vi "OPC UA Client-Write - Multiple Tags.vi"() -> ()   [LabVIEW 2017]
uses:
  <vilib>/OPCUA/controls/NodeId.ctl
  <vilib>/OPCUA/controls/Write Status.ctl
  <vilib>/OPCUA/client/Multiple Write Double Array.vi
  <vilib>/OPCUA/NI OPC UA Client.lvlib
panel:
  out "Temperature Data":dbl[](array[numeric])
  in  "Node Id":string="Process Data.Temperature"
  in  "Stop Button":bool
  in  "Server Endpoint URL":string="opc.tcp://XPS15HPH:49580"
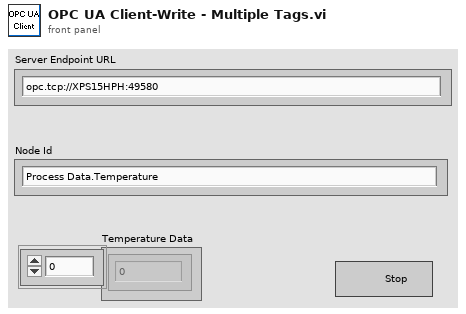
[diagram p1: front panel]
types:
  T1 = cluster{"message mode":enum16{"None", "Sign", "Sign and Encrypt"}, "security":enum16{"Basic256", "Basic128Rsa15"}}
  T2 = typedef "OPC UA Client Refnum.ctl" = refnum<k21>
  T3 = typedef "NodeId.ctl" = string
  T4 = typedef "Write Status.ctl" = u32
  T5 = cluster{"node ID":T3, "value":dbl[], "timestamp (current time)":timestamp, "node status":T4}
  T6 = cluster{"node ID":T3, "value":dbl[], "timestamp (current time)":timestamp, "node status":T4}[]
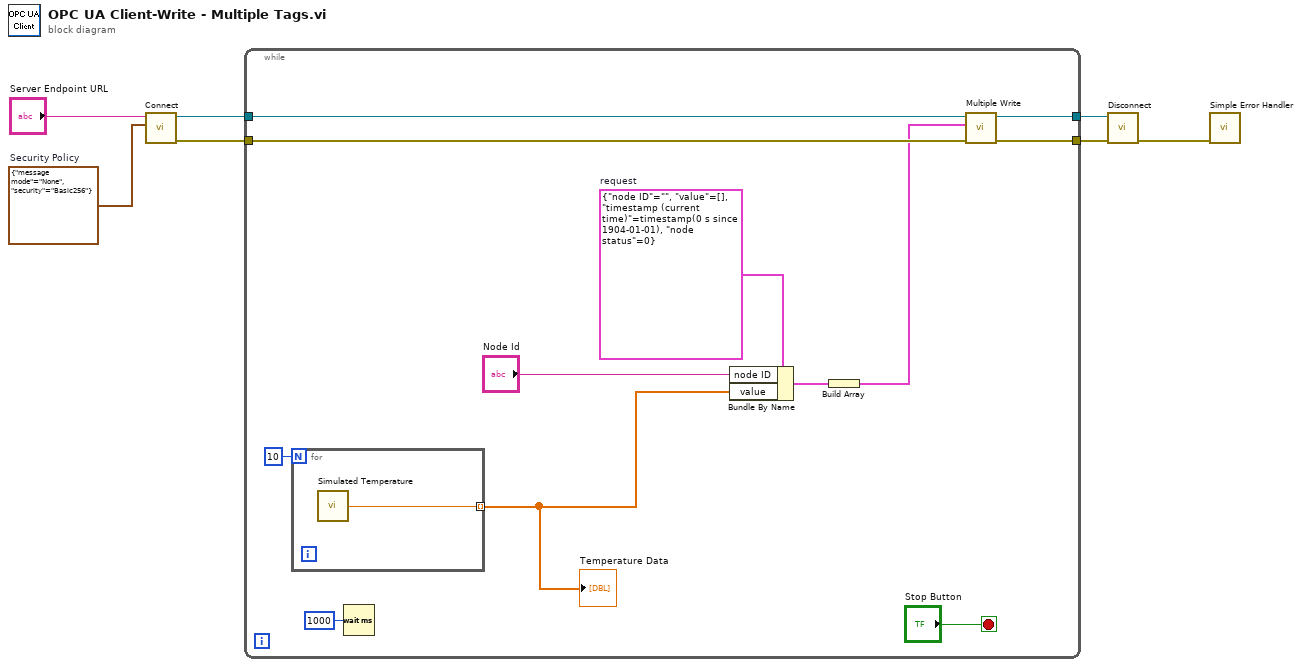
[diagram p0: block diagram]
diagram:
  w1 = T1 {"message mode"=enum."None", "security"=enum."Basic256"}  # Security Policy
  n1 = call <vilib>:"Connect.vi"("security policy"=w1, "server endpoint URL"="Server Endpoint URL") -> ("error out"=w6:errorcluster, "OPC UA client refnum out"=w7:T2)  [unwired: 7 in, 1 out]
  n2 = while {
    tunnel: w7 -> [w17]
    tunnel: w6 -> [w16]
    tunnel: [w15] -> w5
    tunnel: [w14] -> w3
    stop <- "Stop Button" stop-if-true
    w10 = T5 {"node ID"="", "value"=[], "timestamp (current time)"=timestamp(0 s since 1904-01-01), "node status"=0}  # request
    n3 = for {
      N: 10 -> [_]
      tunnel: [w20] -> w9 mode=indexing
      n4 = call "Simulated Temperature.vi"() -> ("Temperature Value"=w20:dbl)  [unwired: 2 in]
    }
    "Temperature Data" <- w9
    n5 = Wait (ms)(milliseconds to wait=u32 1000) -> ()  [unwired: 1 out]
    n6 = Bundle By Name(cluster=w10, "node ID"="Node Id", "value"=w9) -> (w12:T5)
    n7 = Build Array "Build Array"(w12) -> (w8:T6)
    n8 = call-poly <vilib>:"Multiple Write.vi"("error in (no error)"=w16, "requests"=w8, "OPC UA client refnum in"=w17) -> ("error out"=w14:errorcluster, "OPC UA client refnum out"=w15:T2)  [unwired: 5 in, 2 out]
  }
  n9 = call <vilib>:"Disconnect.vi"("error in (no error)"=w3, "OPC UA client refnum in"=w5) -> ("error out"=w4:errorcluster)  [unwired: 9 in]
  n10 = call <vilib>:"Simple Error Handler.vi"("error in (no error)"=w4) -> ()  [unwired: 4 in, 5 out]
